vi "BRig_RT__Case_Exp__State_initTrial__v10.vi"(0 "input_dataCurrent":u16[](array[numeric]), 9 "input_dataBlock":u16[][](array[numeric]), 11 "input_dataTrial":u16[][](array[numeric]), 12 "input_dataExp":u16[](array[numeric])) -> (1 "output_iTrial":u16, 2 "output_nTrial":u16, 3 "output_SolenoidReward":bool, 4 "output_dataCurrent":u16[](array[numeric]), 10 "output_dataBlock":u16[][](array[numeric]), 15 "output_dataTrial":u16[][](array[numeric]))   [LabVIEW 2014]
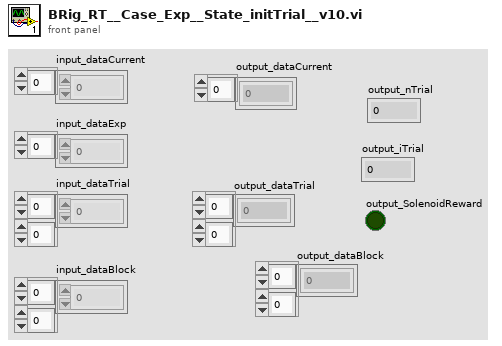
[diagram p1: front panel]
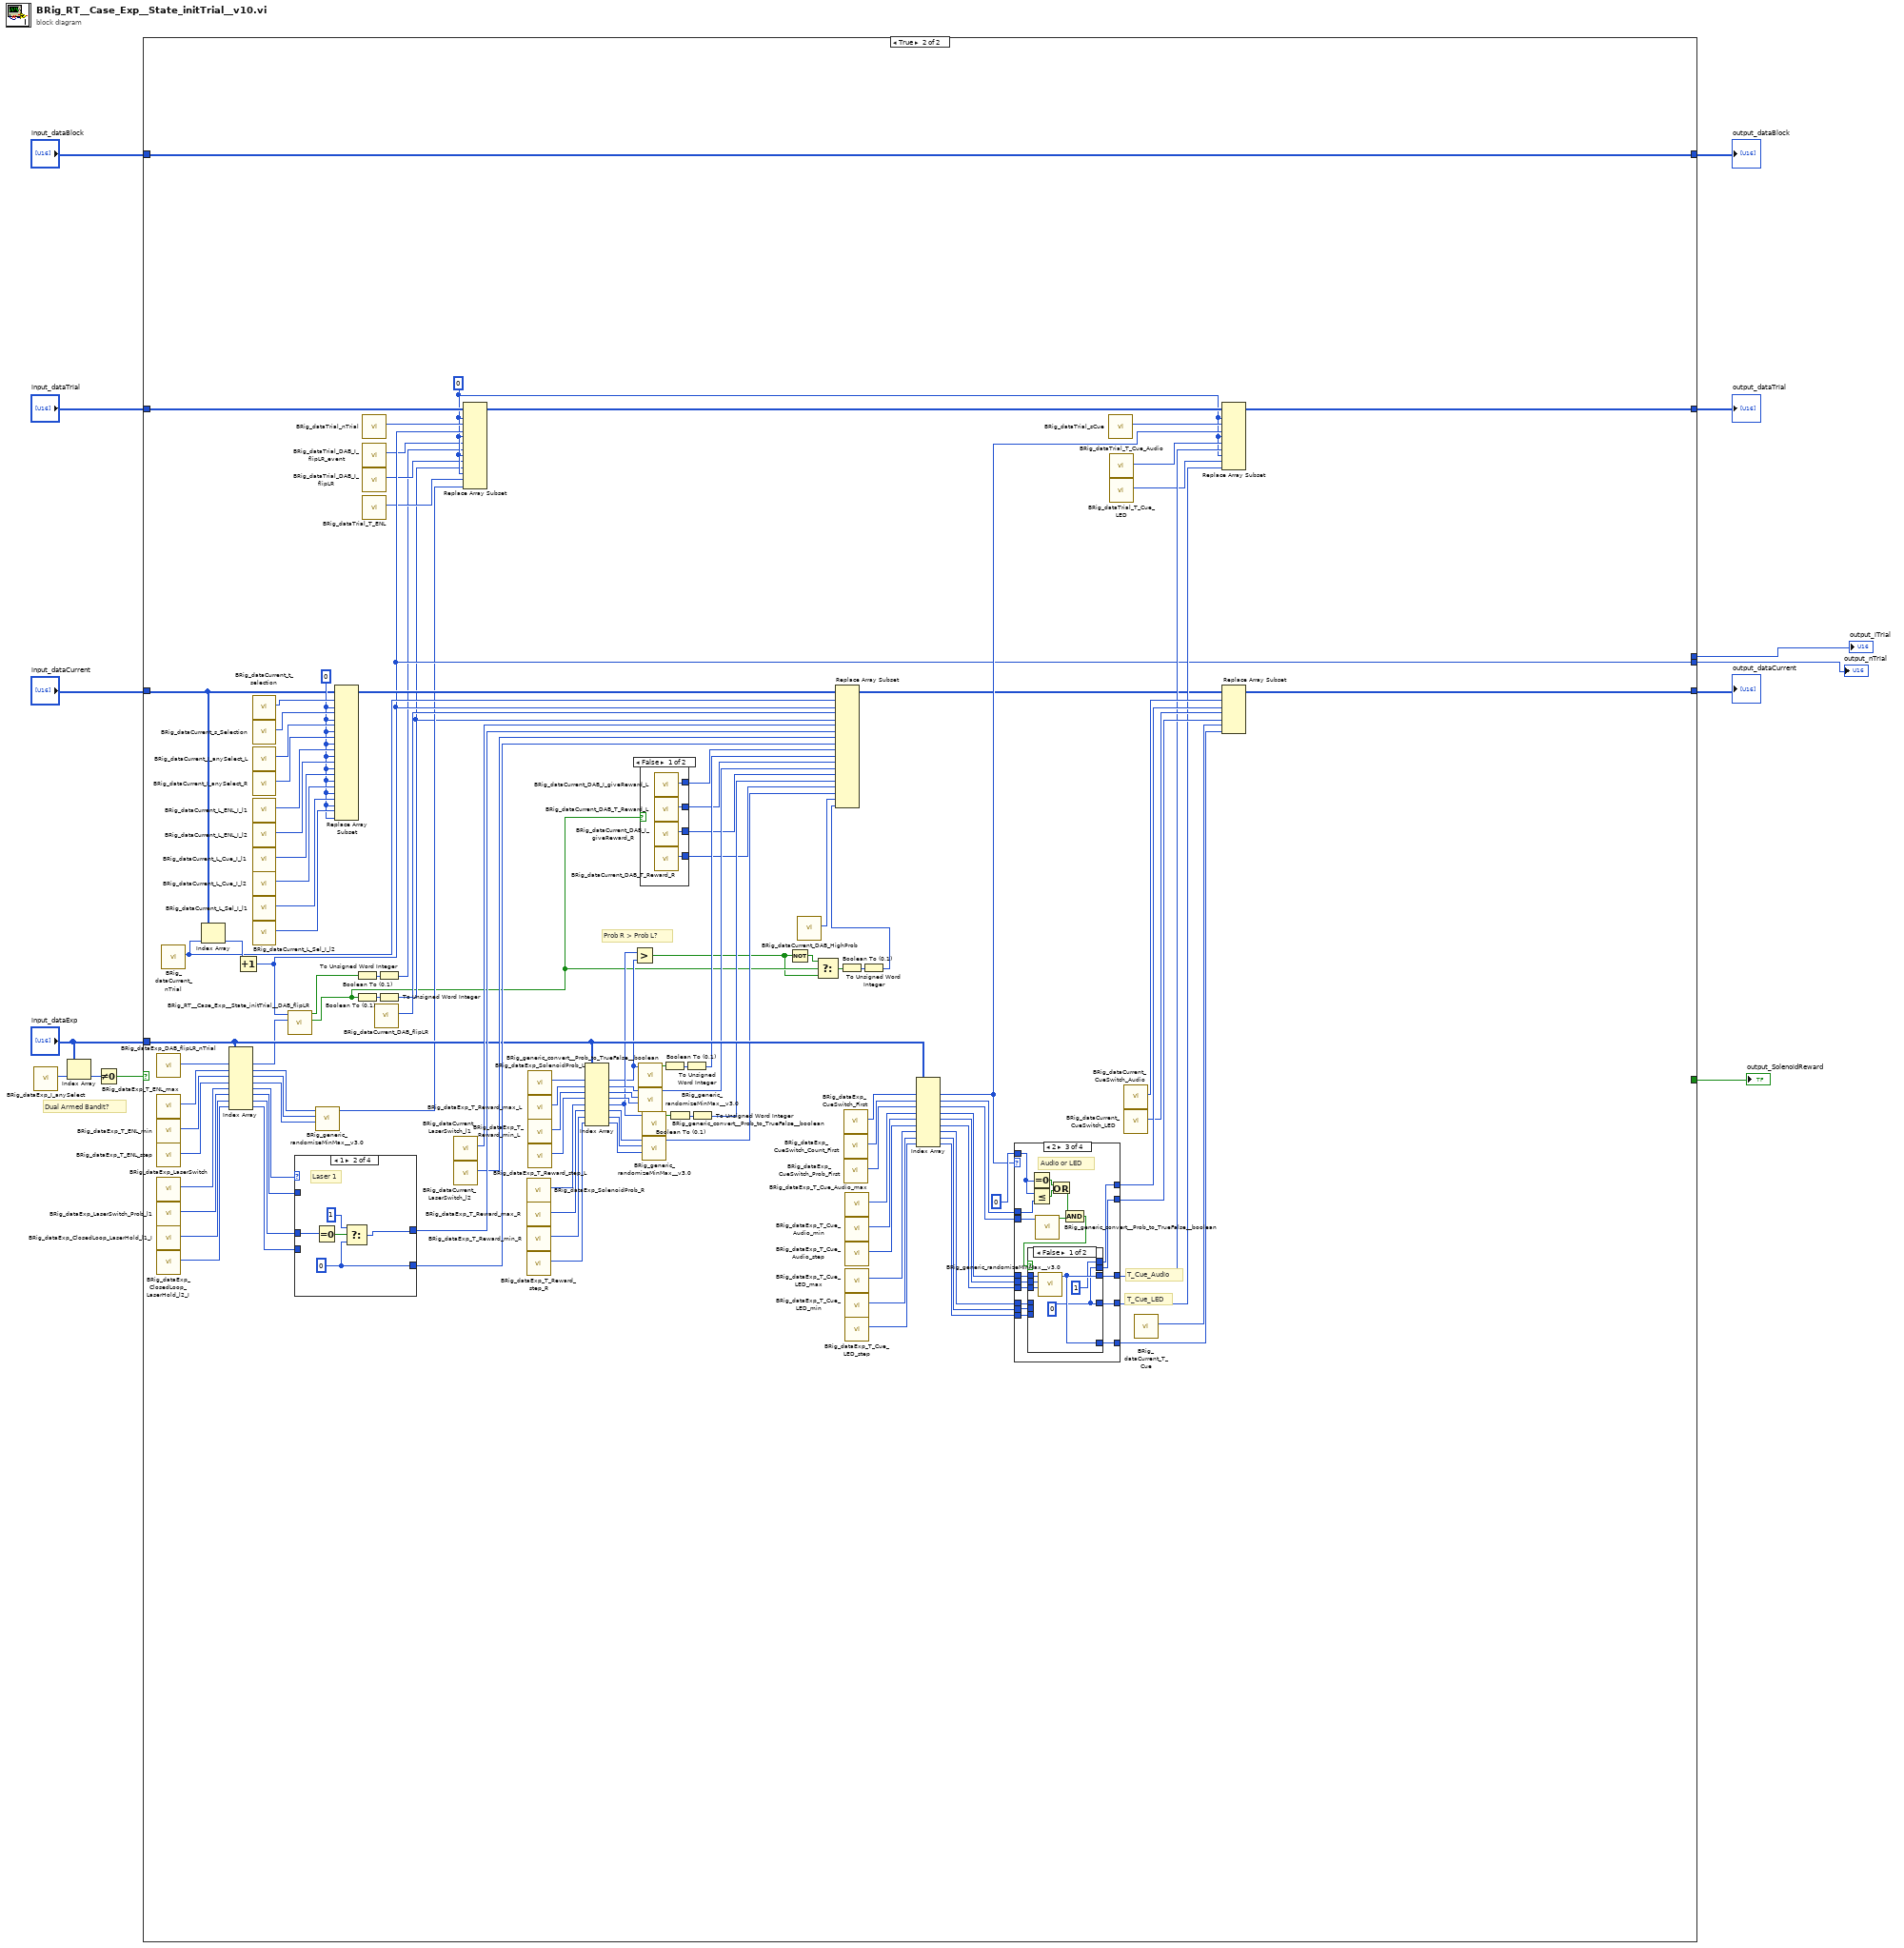
[diagram p0: block diagram]
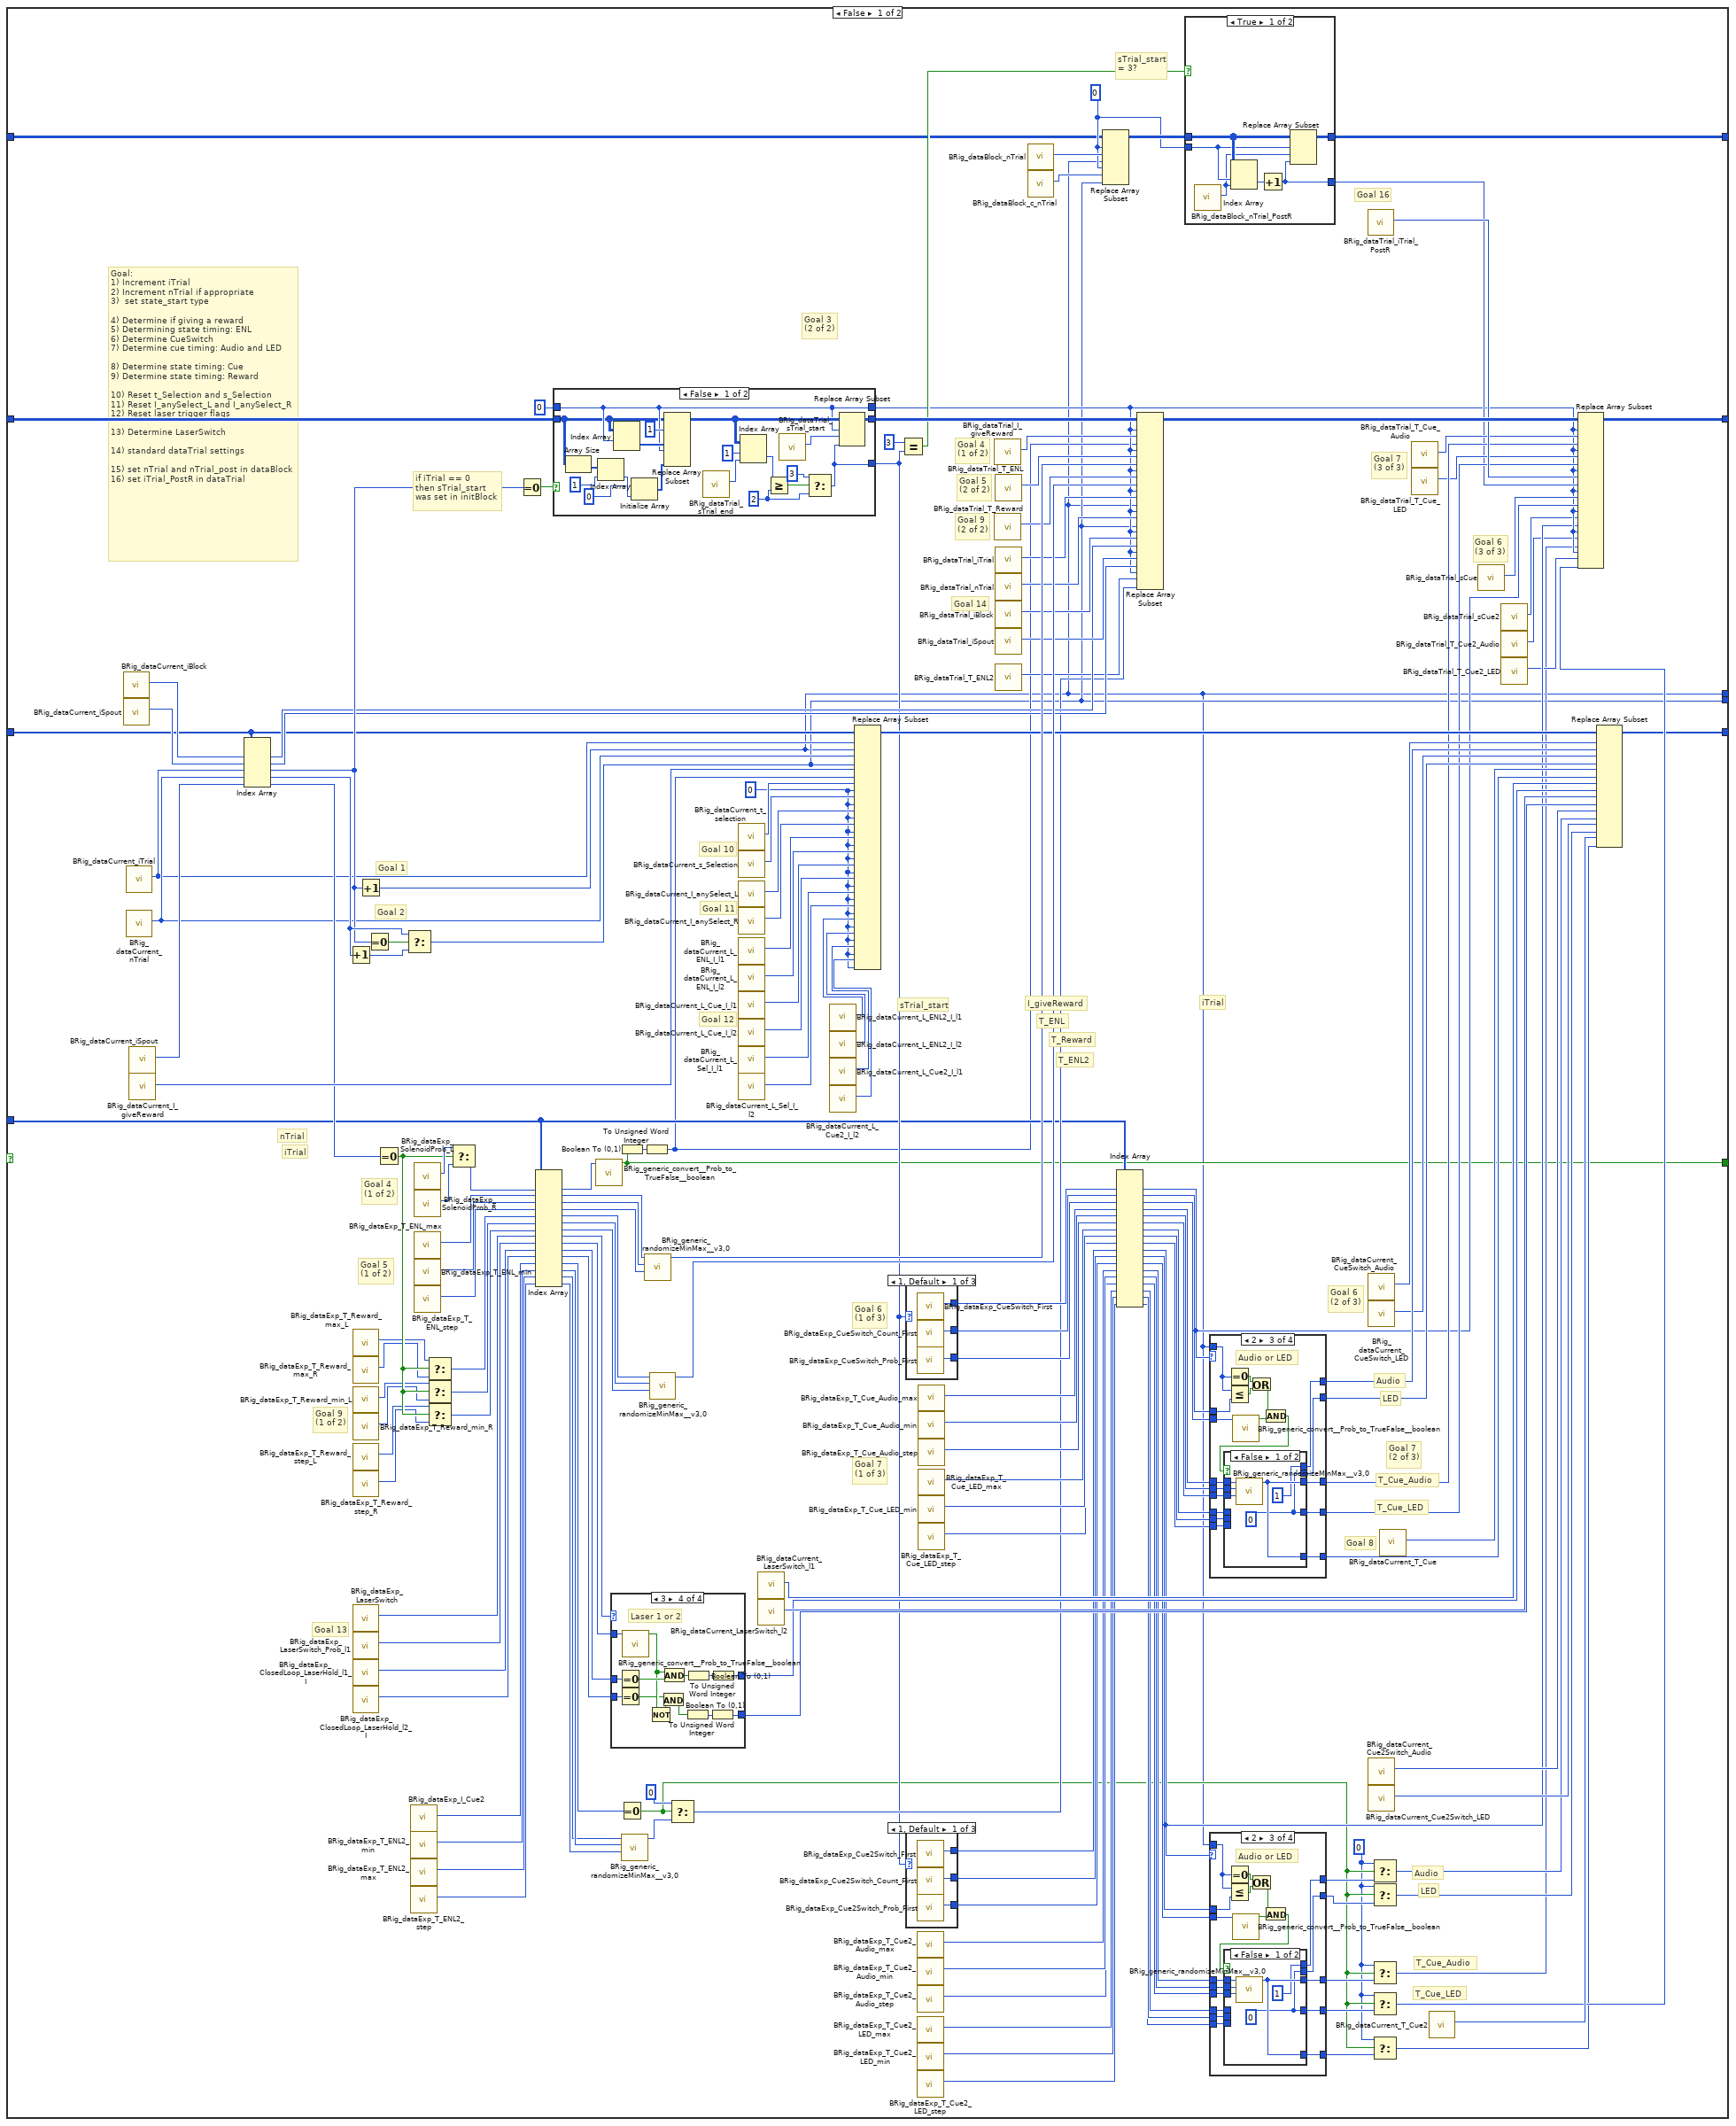
[diagram p2: hidden frame]
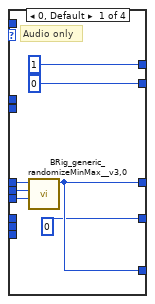
[diagram p3: hidden frame]
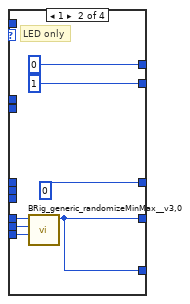
[diagram p4: hidden frame]
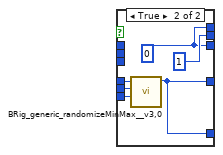
[diagram p5: hidden frame]
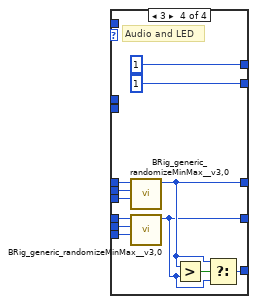
[diagram p6: hidden frame]
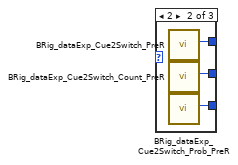
[diagram p7: hidden frame]
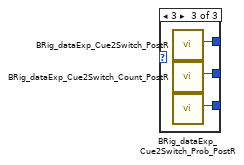
[diagram p8: hidden frame]
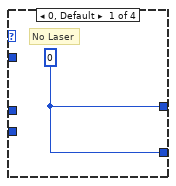
[diagram p10: hidden frame]
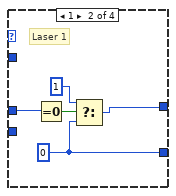
[diagram p11: hidden frame]
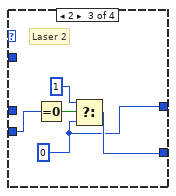
[diagram p12: hidden frame]
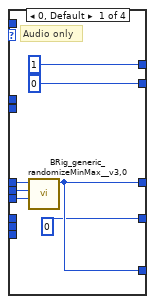
[diagram p13: hidden frame]
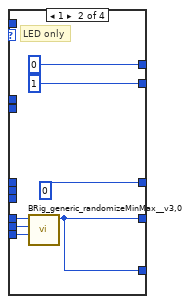
[diagram p14: hidden frame]
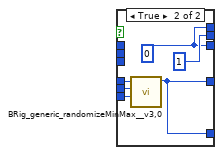
[diagram p15: hidden frame]
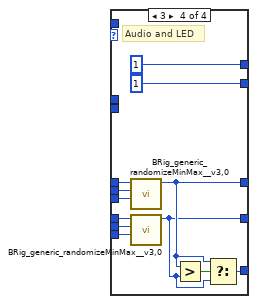
[diagram p16: hidden frame]
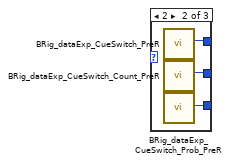
[diagram p17: hidden frame]
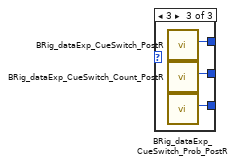
[diagram p18: hidden frame]
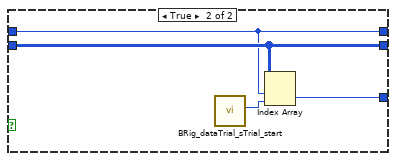
[diagram p19: hidden frame]
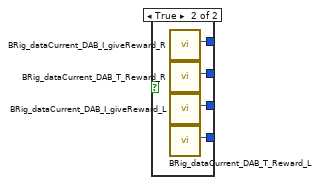
[diagram p20: hidden frame]
diagram:
  # "Dual Armed Bandit?"
  n1 = call "BRig_dataExp_I_anySelect.vi"() -> ("output_I_anySelect"=w13:i32)  [unwired: 11 in]
  n2 = Index Array(array="input_dataExp", index=w13) -> (element=w12:u16)
  n3 = Not Equal To 0?(x=w12) -> (x != 0?=w11:bool)
  n4 = case shown="True" w11 {
    tunnel: "input_dataExp" -> [w24 w421]
    tunnel: "input_dataCurrent" -> [w23 w430]
    tunnel: "input_dataTrial" -> [w22 w433]
    tunnel: "input_dataBlock" -> [w21 w494]
    tunnel: [w20 w494] -> w6
    tunnel: [w19 w447] -> w5
    tunnel: [w18 w448] -> w4
    tunnel: [w17 _] -> w3
    tunnel: [w15 w395] -> w2
    tunnel: [w14 _] -> w1
    frame False {
      w25 = u16 0 ("t")
      w83 = 0 ("disabled index (row)")
      w63 = u16 0 ("new element/subarray")
      # "T_Cue_LED"
      # "T_Cue_Audio"
      # "LED"
      # "Audio"
      # "T_ENL2"
      # "Goal 16"
      # "Goal 6\n(3 of 3)"
      # "iTrial"
      # "sTrial_start\n= 3?"
      # "nTrial"
      # "Goal 14"
      # "Goal 13"
      # "iTrial"
      # "Goal 8"
      # "Goal 7\n(3 of 3)"
      # "Goal 7\n(2 of 3)"
      # "Goal 7\n(1 of 3)"
      # "T_Cue_LED"
      # "T_Cue_Audio"
      # "I_giveReward"
      # "Goal 4\n(1 of 2)"
      # "T_Reward"
      # "Goal 9\n(2 of 2)"
      # "Goal 9\n(1 of 2)"
      # "Goal 12"
      # "Goal 11"
      # "Goal 10"
      # "T_ENL"
      # "sTrial_start"
      # "LED"
      # "Audio"
      # "Goal 6\n(2 of 3)"
      # "Goal 6\n(1 of 3)"
      # "Goal 3\n(2 of 2)"
      # "Goal 5\n(2 of 2)"
      # "Goal 5\n(1 of 2)"
      # "Goal 4\n(1 of 2)"
      # "if iTrial == 0\nthen sTrial_start\nwas set in initBlock"
      # "Goal 2"
      # "Goal 1"
      # "Goal:\n1) Increment iTrial\n2) Increment nTrial if appropriate\n3)  set state_start type\n\n4) Determine if giving a reward\n5) Determining state timing: ENL\n6) Determine CueSwitch\n7) Determine cue timing: Audio and LED\n\n8) Determine state timing: Cue\n9) Determine state timing: Reward\n\n10) Reset t_Selection and s_Selection\n11) Reset I_anySelect_L and I_anySelect_R\n12) Reset laser trigger flags\n\n13) Determine LaserSwitch\n\n14) standard dataTrial settings\n\n15) set nTrial and nTrial_post in dataBlock\n16) set iTrial_PostR in dataTrial"
      n5 = call "BRig_dataCurrent_iBlock.vi"() -> ("output_iBlock"=w99:i32)  [unwired: 11 in]
      n6 = call "BRig_dataCurrent_iSpout.vi"() -> ("output_iSpout"=w98:i32)  [unwired: 11 in]
      n7 = call "BRig_dataCurrent_iTrial.vi"() -> ("output_iTrial"=w80:i32)  [unwired: 11 in]
      n8 = call "BRig_dataCurrent_nTrial.vi"() -> ("output_nTrial"=w81:i32)  [unwired: 11 in]
      n9 = call "BRig_dataCurrent_iSpout.vi"() -> ("output_iSpout"=w90:i32)  [unwired: 11 in]
      n10 = call "BRig_dataCurrent_I_giveReward.vi"() -> ("output_I_giveReward"=w184:i32)  [unwired: 11 in]
      n11 = Index Array(array=w23, index #1=w99, index #2=w98, index #3=w80, index #4=w81, index #5=w90) -> (element #1=w108:u16, element #2=w107:u16, element #3=w121:u16, element #4=w188:u16, element #5=w89:u16)
      n12 = Increment(x=w188) -> (x+1=w187:u16)
      n13 = call "BRig_dataExp_T_Reward_max_L.vi"() -> ("output_T_Reward_max_L"=w152:i32)  [unwired: 11 in]
      n14 = call "BRig_dataExp_T_Reward_max_R.vi"() -> ("output_T_Reward_max_R"=w151:i32)  [unwired: 11 in]
      n15 = call "BRig_dataExp_T_Reward_min_L.vi"() -> ("output_Tcycle_Reward_min_L"=w150:i32)  [unwired: 11 in]
      n16 = call "BRig_dataExp_T_Reward_min_R.vi"() -> ("output_T_Reward_min_R"=w149:i32)  [unwired: 11 in]
      n17 = call "BRig_dataExp_T_Reward_step_L.vi"() -> ("output_T_Reward_step_L"=w148:i32)  [unwired: 11 in]
      n18 = call "BRig_dataExp_T_Reward_step_R.vi"() -> ("output_T_Reward_step_R"=w147:i32)  [unwired: 11 in]
      n19 = call "BRig_dataExp_LaserSwitch.vi"() -> ("output_LaserSwitch"=w120:i32)  [unwired: 11 in]
      n20 = call "BRig_dataExp_LaserSwitch_Prob_l1.vi"() -> ("output_LaserSwitch_Probability_L1"=w119:i32)  [unwired: 11 in]
      n21 = call "BRig_dataExp_ClosedLoop_LaserHold_l1_I.vi"() -> ("output_CloseLoop_LaserHold_l1_I"=w95:i32)  [unwired: 11 in]
      n22 = call "BRig_dataExp_ClosedLoop_LaserHold_l2_I.vi"() -> ("output_CloseLoop_LaserHold_l2_I"=w94:i32)  [unwired: 11 in]
      n23 = Increment(x=w121) -> (x+1=w14:u16)
      n24 = Equal To 0?(x=w121) -> (x = 0?=w186:bool)
      n25 = Equal To 0?(x=w89) -> (x = 0?=w153:bool)
      n26 = Select(t=w188, s=w186, f=w187) -> (s? t:f=w15:u16)
      n27 = call "BRig_dataExp_I_Cue2.vi"() -> ("output_I_Cue2"=w79:i32)  [unwired: 11 in]
      n28 = call "BRig_dataExp_T_ENL2_min.vi"() -> ("output_T_ENL2_min"=w78:i32)  [unwired: 11 in]
      n29 = call "BRig_dataExp_T_ENL2_max.vi"() -> ("output_T_ENL2_max"=w77:i32)  [unwired: 11 in]
      n30 = call "BRig_dataExp_T_ENL2_step.vi"() -> ("output_T_ENL2_step"=w76:i32)  [unwired: 11 in]
      n31 = call "BRig_dataExp_SolenoidProb_L.vi"() -> ("output_SolenoidProbability_L"=w183:i32)  [unwired: 11 in]
      n32 = call "BRig_dataExp_SolenoidProb_R.vi"() -> ("output_SolenoidProbability_R"=w182:i32)  [unwired: 11 in]
      n33 = call "BRig_dataExp_T_ENL_max.vi"() -> ("output_T_ENL_max"=w177:i32)  [unwired: 11 in]
      n34 = call "BRig_dataExp_T_ENL_min.vi"() -> ("output_T_ENL_min"=w178:i32)  [unwired: 11 in]
      n35 = call "BRig_dataExp_T_ENL_step.vi"() -> ("output_T_ENL_step"=w179:i32)  [unwired: 11 in]
      n36 = Select(t=w152, s=w153, f=w151) -> (s? t:f=w146:i32)
      n37 = Select(t=w150, s=w153, f=w149) -> (s? t:f=w145:i32)
      n38 = Select(t=w148, s=w153, f=w147) -> (s? t:f=w144:i32)
      n39 = Select(t=w183, s=w153, f=w182) -> (s? t:f=w181:i32)
      n40 = Equal To 0?(x=w121) -> (x = 0?=w185:bool)
      n41 = Index Array(array=w24, index #1=w181, index #2=w177, index #3=w178, index #4=w179, index #5=w146, index #6=w145, index #7=w144, index #8=w120, index #9=w119, index #10=w95, index #11=w94, index #12=w79, index #13=w78, index #14=w77, index #15=w76) -> (element #1=w180:u16, element #2=w176:u16, element #3=w175:u16, element #4=w174:u16, element #5=w143:u16, element #6=w142:u16, element #7=w141:u16, element #8=w118:u16, element #9=w117:u16, element #10=w93:u16, element #11=w92:u16, element #12=w73:u16, element #13=w72:u16, element #14=w71:u16, element #15=w70:u16)
      n42 = case shown="False" w185 {
        tunnel: w22 -> [w358 w375]
        tunnel: [w369 w375] -> w173
        tunnel: 0 -> [w359 w374]
        tunnel: [w359 w374] -> w37
        tunnel: [w365 w372] -> w62
        frame False {
          w366 = u16 2 ("y")
          n43 = Array Size(array=w358) -> (size(s)=w357:i32[])
          n44 = Index Array(array=w357, index=1) -> (element=w355:i32)
          n45 = Index Array(array=w358, index (row)=w359) -> (element=w362:u16[])  [unwired: 1 in]
          n46 = Initialize Array(u16 0 ("index"), w355) -> (w353:u16[])
          n47 = Replace Array Subset(array=w358, new element #1=w362, index (row) #1=1 ("index (row)"), new element #2=w353, index (row) #2=w359) -> (w360:u16[][])  [unwired: 2 in]
          n48 = call "BRig_dataTrial_sTrial_end.vi"() -> ("output_sTrial_end"=w371:i32)  [unwired: 11 in]
          n49 = Index Array(array=w360, index (row)=1 ("disabled index (row)"), index (col)=w371) -> (element=w370:u16)
          n50 = Greater Or Equal?(x=w370, y=w366) -> (x >= y?=w368:bool)
          n51 = call "BRig_dataTrial_sTrial_start.vi"() -> ("output_sTrial_start"=w364:i32)  [unwired: 11 in]
          n52 = Select(t=u16 3 ("y"), s=w368, f=w366) -> (s? t:f=w365:u16)
          n53 = Replace Array Subset(array=w360, new element=w365, index (row)=w359, index (col)=w364) -> (w369:u16[][])
        }
        frame True {
          n54 = call "BRig_dataTrial_sTrial_start.vi"() -> ("output_sTrial_start"=w373:i32)  [unwired: 11 in]
          n55 = Index Array(array=w375, index (row)=w374, index (col)=w373) -> (element=w372:u16)
        }
      }
      n56 = call "BRig_generic_convert__Prob_to_TrueFalse__boolean.vi"("input_probability_u16"=w180) -> ("output_TF"=w17:bool)  [unwired: 10 in]
      n57 = case shown="3" w118 {
        tunnel: [w263 w264 w269 w283] -> w115
        tunnel: [w263 w265 w270 w282] -> w114
        tunnel: w117 -> [_ _ _ w286]
        tunnel: w93 -> [_ w268 _ w281]
        tunnel: w92 -> [_ _ w271 w280]
        frame 0, Default {
          w263 = u16 0
          # "No Laser"
        }
        frame 1 {
          w265 = u16 0
          # "Laser 1"
          n58 = Equal To 0?(x=w268) -> (x = 0?=w267:bool)
          n59 = Select(t=u16 1, s=w267, f=w265) -> (s? t:f=w264:u16)
        }
        frame 2 {
          w269 = u16 0
          # "Laser 2"
          n60 = Equal To 0?(x=w271) -> (x = 0?=w273:bool)
          n61 = Select(t=u16 1, s=w273, f=w269) -> (s? t:f=w270:u16)
        }
        frame 3 {
          # "Laser 1 or 2"
          n62 = Equal To 0?(x=w281) -> (x = 0?=w279:bool)
          n63 = Equal To 0?(x=w280) -> (x = 0?=w275:bool)
          n64 = call "BRig_generic_convert__Prob_to_TrueFalse__boolean.vi"("input_probability_u16"=w286) -> ("output_TF"=w278:bool)  [unwired: 10 in]
          n65 = Not(x=w278) -> (.not. x?=w276:bool)
          n66 = And(x=w275, y=w276) -> (x .and. y?=w274:bool)
          n67 = And(x=w278, y=w279) -> (x .and. y?=w277:bool)
          n68 = Boolean To (0,1)(Boolean=w274) -> (0, 1=w285:i16)
          n69 = Boolean To (0,1)(Boolean=w277) -> (0, 1=w284:i16)
          n70 = To Unsigned Word Integer(number=w285) -> (unsigned 16bit integer=w282:u16)
          n71 = To Unsigned Word Integer(number=w284) -> (unsigned 16bit integer=w283:u16)
        }
      }
      n72 = Boolean To (0,1)(Boolean=w17) -> (0, 1=w189:i16)
      n73 = Equal To 0?(x=w73) -> (x = 0?=w26:bool)
      n74 = call "BRig_generic_randomizeMinMax__v3,0.vi"("Input_Increment"=w70, "Input_Min"=w72, "Input_Max"=w71) -> ("Output"=w75:u16)  [unwired: 8 in]
      n75 = To Unsigned Word Integer(number=w189) -> (unsigned 16bit integer=w16:u16)
      n76 = call "BRig_generic_randomizeMinMax__v3,0.vi"("Input_Increment"=w174, "Input_Min"=w175, "Input_Max"=w176) -> ("Output"=w171:u16)  [unwired: 8 in]
      n77 = call "BRig_generic_randomizeMinMax__v3,0.vi"("Input_Increment"=w141, "Input_Min"=w142, "Input_Max"=w143) -> ("Output"=w139:u16)  [unwired: 8 in]
      n78 = Select(t=u16 0, s=w26, f=w75) -> (s? t:f=w68:u16)
      n79 = call "BRig_dataCurrent_t_selection.vi"() -> ("output_t_selection"=w163:i32)  [unwired: 11 in]
      n80 = call "BRig_dataCurrent_s_Selection.vi"() -> ("output_s_Selection"=w162:i32)  [unwired: 11 in]
      n81 = call "BRig_dataCurrent_I_anySelect_L.vi"() -> ("output_IanySelect_L"=w161:i32)  [unwired: 11 in]
      n82 = call "BRig_dataCurrent_I_anySelect_R.vi"() -> ("output_IanySelect_R"=w160:i32)  [unwired: 11 in]
      n83 = call "BRig_dataCurrent_L_ENL_I_l1.vi"() -> ("output_L_ENL_I_l1"=w159:i32)  [unwired: 11 in]
      n84 = call "BRig_dataCurrent_L_ENL_I_l2.vi"() -> ("output_L_ENL_I_l2"=w158:i32)  [unwired: 11 in]
      n85 = call "BRig_dataCurrent_L_Cue_I_l1.vi"() -> ("output_L_Cue_I_l1"=w157:i32)  [unwired: 11 in]
      n86 = call "BRig_dataCurrent_L_Cue_I_l2.vi"() -> ("output_L_Cue_I_l2"=w156:i32)  [unwired: 11 in]
      n87 = call "BRig_dataCurrent_L_Sel_I_l1.vi"() -> ("output_L_Sel_I_l1"=w155:i32)  [unwired: 11 in]
      n88 = call "BRig_dataCurrent_L_Sel_I_l2.vi"() -> ("output_L_Sel_I_l2"=w154:i32)  [unwired: 11 in]
      n89 = call "BRig_dataCurrent_LaserSwitch_l1.vi"() -> ("output_LaserSwitch_l1"=w113:i32)  [unwired: 11 in]
      n90 = call "BRig_dataCurrent_LaserSwitch_l2.vi"() -> ("output_LaserSwitch_l2"=w116:i32)  [unwired: 11 in]
      n91 = call "BRig_dataCurrent_L_ENL2_I_l1.vi"() -> ("output_L_ENL2_I_l1"=w67:i32)  [unwired: 11 in]
      n92 = call "BRig_dataCurrent_L_ENL2_I_l2.vi"() -> ("output_L_ENL2_I_l2"=w66:i32)  [unwired: 11 in]
      n93 = call "BRig_dataCurrent_L_Cue2_I_l1.vi"() -> ("output_L_Cue2_I_l1"=w65:i32)  [unwired: 11 in]
      n94 = call "BRig_dataCurrent_L_Cue2_I_l2.vi"() -> ("output_L_Cue2_I_l2"=w64:i32)  [unwired: 11 in]
      n95 = Replace Array Subset(array=w23, new element #1=w14, index #1=w80, new element #2=w15, index #2=w81, new element #3=w16, index #3=w184, new element #4=w63, index #4=w163, new element #5=w63, index #5=w162, new element #6=w63, index #6=w161, new element #7=w63, index #7=w160, new element #8=w63, index #8=w159, new element #9=w63, index #9=w158, new element #10=w63, index #10=w157, new element #11=w63, index #11=w156, new element #12=w63, index #12=w155, new element #13=w63, index #13=w154, new element #14=w63, index #14=w67, new element #15=w63, index #15=w66, new element #16=w63, index #16=w65, new element #17=w63, index #17=w64) -> (w106:u16[])
      n96 = Equal?(x=u16 3 ("y"), y=w62) -> (x = y?=w84:bool)
      n97 = case shown="1, Default" w62 {
        tunnel: [w346 w347 w352] -> w170
        tunnel: [w345 w348 w351] -> w169
        tunnel: [w344 w349 w350] -> w168
        frame 1, Default {
          n98 = call "BRig_dataExp_CueSwitch_First.vi"() -> ("output_CueSwitch_First"=w346:i32)  [unwired: 11 in]
          n99 = call "BRig_dataExp_CueSwitch_Count_First.vi"() -> ("output_CueSwitch_Count_First"=w345:i32)  [unwired: 11 in]
          n100 = call "BRig_dataExp_CueSwitch_Prob_First.vi"() -> ("output_CueSwitch_Prob_First"=w344:i32)  [unwired: 11 in]
        }
        frame 2 {
          n101 = call "BRig_dataExp_CueSwitch_PreR.vi"() -> ("output_CueSwitch_PreR"=w347:i32)  [unwired: 11 in]
          n102 = call "BRig_dataExp_CueSwitch_Count_PreR.vi"() -> ("output_CueSwitch_Count_PreR"=w348:i32)  [unwired: 11 in]
          n103 = call "BRig_dataExp_CueSwitch_Prob_PreR.vi"() -> ("output_CueSwitch_Prob_PreR"=w349:i32)  [unwired: 11 in]
        }
        frame 3 {
          n104 = call "BRig_dataExp_CueSwitch_PostR.vi"() -> ("output_CueSwitch_PostR"=w352:i32)  [unwired: 11 in]
          n105 = call "BRig_dataExp_CueSwitch_Count_PostR.vi"() -> ("output_CueSwitch_Count_PostR"=w351:i32)  [unwired: 11 in]
          n106 = call "BRig_dataExp_CueSwitch_Prob_PostR.vi"() -> ("output_CueSwitch_Prob_PostR"=w350:i32)  [unwired: 11 in]
        }
      }
      n107 = case shown="1, Default" w62 {
        tunnel: [w249 w252 w255] -> w61
        tunnel: [w248 w251 w254] -> w60
        tunnel: [w247 w250 w253] -> w59
        frame 1, Default {
          n108 = call "BRig_dataExp_Cue2Switch_First.vi"() -> ("output_Cue2Switch_First"=w249:i32)  [unwired: 11 in]
          n109 = call "BRig_dataExp_Cue2Switch_Count_First.vi"() -> ("output_Cue2Switch_Count_First"=w248:i32)  [unwired: 11 in]
          n110 = call "BRig_dataExp_Cue2Switch_Prob_First.vi"() -> ("output_Cue2Switch_Prob_First"=w247:i32)  [unwired: 11 in]
        }
        frame 2 {
          n111 = call "BRig_dataExp_Cue2Switch_PreR.vi"() -> ("output_Cue2Switch_PreR"=w252:i32)  [unwired: 11 in]
          n112 = call "BRig_dataExp_Cue2Switch_Count_PreR.vi"() -> ("output_Cue2Switch_Count_PreR"=w251:i32)  [unwired: 11 in]
          n113 = call "BRig_dataExp_Cue2Switch_Prob_PreR.vi"() -> ("output_Cue2Switch_Prob_PreR"=w250:i32)  [unwired: 11 in]
        }
        frame 3 {
          n114 = call "BRig_dataExp_Cue2Switch_PostR.vi"() -> ("output_Cue2Switch_PostR"=w255:i32)  [unwired: 11 in]
          n115 = call "BRig_dataExp_Cue2Switch_Count_PostR.vi"() -> ("output_Cue2Switch_Count_PostR"=w254:i32)  [unwired: 11 in]
          n116 = call "BRig_dataExp_Cue2Switch_Prob_PostR.vi"() -> ("output_Cue2Switch_Prob_PostR"=w253:i32)  [unwired: 11 in]
        }
      }
      n117 = call "BRig_dataExp_T_Cue2_Audio_max.vi"() -> ("output_T_Cue2_Audio_max"=w58:i32)  [unwired: 11 in]
      n118 = call "BRig_dataExp_T_Cue2_Audio_min.vi"() -> ("output_T_Cue2_Audio_min"=w57:i32)  [unwired: 11 in]
      n119 = call "BRig_dataExp_T_Cue2_Audio_step.vi"() -> ("output_T_Cue2_Audio_step"=w56:i32)  [unwired: 11 in]
      n120 = call "BRig_dataExp_T_Cue2_LED_max.vi"() -> ("output_T_Cue2_LED_max"=w55:i32)  [unwired: 11 in]
      n121 = call "BRig_dataExp_T_Cue2_LED_min.vi"() -> ("output_T_Cue2_LED_min"=w54:i32)  [unwired: 11 in]
      n122 = call "BRig_dataExp_T_Cue2_LED_step.vi"() -> ("output_T_Cue2_LED_step"=w53:i32)  [unwired: 11 in]
      n123 = call "BRig_dataExp_T_Cue_Audio_max.vi"() -> ("output_T_Cue_Audio_max"=w137:i32)  [unwired: 11 in]
      n124 = call "BRig_dataExp_T_Cue_Audio_min.vi"() -> ("output_T_Cue_Audio_min"=w136:i32)  [unwired: 11 in]
      n125 = call "BRig_dataExp_T_Cue_Audio_step.vi"() -> ("output_T_Cue_Audio_step"=w135:i32)  [unwired: 11 in]
      n126 = call "BRig_dataExp_T_Cue_LED_max.vi"() -> ("output_T_Cue_LED_max"=w134:i32)  [unwired: 11 in]
      n127 = call "BRig_dataExp_T_Cue_LED_min.vi"() -> ("output_T_Cue_LED_min"=w133:i32)  [unwired: 11 in]
      n128 = call "BRig_dataExp_T_Cue_LED_step.vi"() -> ("output_T_Cue_LED_step"=w132:i32)  [unwired: 11 in]
      n129 = call "BRig_dataTrial_I_giveReward.vi"() -> ("output_I_giveReward"=w138:i32)  [unwired: 11 in]
      n130 = call "BRig_dataTrial_T_Reward.vi"() -> ("output_T_Reward"=w140:i32)  [unwired: 11 in]
      n131 = call "BRig_dataTrial_T_ENL.vi"() -> ("output_T_ENL"=w172:i32)  [unwired: 11 in]
      n132 = call "BRig_dataTrial_iTrial.vi"() -> ("output_iTrial"=w112:i32)  [unwired: 11 in]
      n133 = call "BRig_dataTrial_nTrial.vi"() -> ("output_nTrial"=w111:i32)  [unwired: 11 in]
      n134 = call "BRig_dataTrial_iBlock.vi"() -> ("output_iBlock"=w110:i32)  [unwired: 11 in]
      n135 = call "BRig_dataTrial_iSpout.vi"() -> ("output_iSpout"=w109:i32)  [unwired: 11 in]
      n136 = call "BRig_dataTrial_T_ENL2.vi"() -> ("output_T_ENL2"=w69:i32)  [unwired: 11 in]
      n137 = call "BRig_dataBlock_nTrial.vi"() -> ("output_nTrial"=w86:i32)  [unwired: 11 in]
      n138 = call "BRig_dataBlock_c_nTrial.vi"() -> ("output_c_nTrial"=w85:i32)  [unwired: 11 in]
      n139 = Replace Array Subset(array=w21, new element #1=w14, index (row) #1=w83, index (col) #1=w86, new element #2=w15, index (row) #2=w83, index (col) #2=w85) -> (w87:u16[][])
      n140 = Index Array(array=w24, index #1=w170, index #2=w169, index #3=w168, index #4=w137, index #5=w136, index #6=w135, index #7=w134, index #8=w133, index #9=w132, index #10=w61, index #11=w60, index #12=w59, index #13=w58, index #14=w57, index #15=w56, index #16=w55, index #17=w54, index #18=w53) -> (element #1=w96:u16, element #2=w131:u16, element #3=w130:u16, element #4=w129:u16, element #5=w128:u16, element #6=w127:u16, element #7=w126:u16, element #8=w125:u16, element #9=w124:u16, element #10=w36:u16, element #11=w52:u16, element #12=w51:u16, element #13=w50:u16, element #14=w49:u16, element #15=w48:u16, element #16=w47:u16, element #17=w46:u16, element #18=w45:u16)
      n141 = Replace Array Subset(array=w173, new element #1=w16, index (row) #1=w37, index (col) #1=w138, new element #2=w171, index (row) #2=w37, index (col) #2=w172, new element #3=w139, index (row) #3=w37, index (col) #3=w140, new element #4=w14, index (row) #4=w37, index (col) #4=w112, new element #5=w15, index (row) #5=w37, index (col) #5=w111, new element #6=w108, index (row) #6=w37, index (col) #6=w110, new element #7=w107, index (row) #7=w37, index (col) #7=w109, new element #8=w68, index (row) #8=w37, index (col) #8=w69) -> (w105:u16[][])
      n142 = case shown="True" w84 {
        tunnel: w87 -> [w261 w262]
        tunnel: [w259 w262] -> w20
        tunnel: [w256 _] -> w82
        tunnel: w83 -> [w258 _]
        frame True {
          n143 = call "BRig_dataBlock_nTrial_PostR.vi"() -> ("output_nTrial_PostR"=w257:i32)  [unwired: 11 in]
          n144 = Index Array(array=w261, index (row)=w258, index (col)=w257) -> (element=w260:u16)
          n145 = Increment(x=w260) -> (x+1=w256:u16)
          n146 = Replace Array Subset(array=w261, new element=w256, index (row)=w258, index (col)=w257) -> (w259:u16[][])
        }
        frame False {
        }
      }
      n147 = case shown="2" w96 {
        tunnel: [u16 1 u16 0 w305 u16 1] -> w166
        tunnel: [u16 0 u16 1 w304 u16 1] -> w164
        tunnel: w131 -> [_ _ w318 _]
        tunnel: w130 -> [_ _ w315 _]
        tunnel: w129 -> [w291 _ w311 w341]
        tunnel: w128 -> [w290 _ w310 w340]
        tunnel: w127 -> [w289 _ w309 w339]
        tunnel: w126 -> [_ w298 w303 w338]
        tunnel: w125 -> [_ w297 w302 w337]
        tunnel: w124 -> [_ w296 w301 w336]
        tunnel: [w288 u16 0 ("Output") w308 w334] -> w103
        tunnel: [u16 0 ("Output") w295 w306 w333] -> w102
        tunnel: [w288 w295 w307 w332] -> w122
        tunnel: w14 -> [_ _ w319 _]
        frame 0, Default {
          # "Audio only"
          n148 = call "BRig_generic_randomizeMinMax__v3,0.vi"("Input_Increment"=w289, "Input_Min"=w290, "Input_Max"=w291) -> ("Output"=w288:u16)  [unwired: 8 in]
        }
        frame 1 {
          # "LED only"
          n149 = call "BRig_generic_randomizeMinMax__v3,0.vi"("Input_Increment"=w296, "Input_Min"=w297, "Input_Max"=w298) -> ("Output"=w295:u16)  [unwired: 8 in]
        }
        frame 2 {
          # "Audio or LED"
          n150 = Equal To 0?(x=w319) -> (x = 0?=w317:bool)
          n151 = Less Or Equal?(x=w319, y=w318) -> (x <= y?=w316:bool)
          n152 = call "BRig_generic_convert__Prob_to_TrueFalse__boolean.vi"("input_probability_u16"=w315) -> ("output_TF"=w314:bool)  [unwired: 10 in]
          n153 = Or(x=w317, y=w316) -> (x .or. y?=w313:bool)
          n154 = And(x=w313, y=w314) -> (x .and. y?=w312:bool)
          n155 = case shown="False" w312 {
            tunnel: w311 -> [w325 _]
            tunnel: w310 -> [w324 _]
            tunnel: w309 -> [w323 _]
            tunnel: [w322 w326] -> w308
            tunnel: [w322 w328] -> w307
            tunnel: [w320 w328] -> w306
            tunnel: [u16 1 w326] -> w305
            tunnel: [w320 u16 1] -> w304
            tunnel: w303 -> [_ w331]
            tunnel: w302 -> [_ w330]
            tunnel: w301 -> [_ w329]
            frame False {
              w320 = u16 0
              n156 = call "BRig_generic_randomizeMinMax__v3,0.vi"("Input_Increment"=w323, "Input_Min"=w324, "Input_Max"=w325) -> ("Output"=w322:u16)  [unwired: 8 in]
            }
            frame True {
              w326 = u16 0
              n157 = call "BRig_generic_randomizeMinMax__v3,0.vi"("Input_Increment"=w329, "Input_Min"=w330, "Input_Max"=w331) -> ("Output"=w328:u16)  [unwired: 8 in]
            }
          }
        }
        frame 3 {
          # "Audio and LED"
          n158 = call "BRig_generic_randomizeMinMax__v3,0.vi"("Input_Increment"=w339, "Input_Min"=w340, "Input_Max"=w341) -> ("Output"=w334:u16)  [unwired: 8 in]
          n159 = call "BRig_generic_randomizeMinMax__v3,0.vi"("Input_Increment"=w336, "Input_Min"=w337, "Input_Max"=w338) -> ("Output"=w333:u16)  [unwired: 8 in]
          n160 = Greater?(x=w334, y=w333) -> (0:w335:bool)
          n161 = Select(t=w334, s=w335, f=w333) -> (s? t:f=w332:u16)
        }
      }
      n162 = case shown="2" w36 {
        tunnel: [u16 1 u16 0 w208 u16 1] -> w43
        tunnel: [u16 0 u16 1 w207 u16 1] -> w44
        tunnel: w52 -> [_ _ w221 _]
        tunnel: w51 -> [_ _ w218 _]
        tunnel: w50 -> [w194 _ w214 w244]
        tunnel: w49 -> [w193 _ w213 w243]
        tunnel: w48 -> [w192 _ w212 w242]
        tunnel: w47 -> [_ w201 w206 w241]
        tunnel: w46 -> [_ w200 w205 w240]
        tunnel: w45 -> [_ w199 w204 w239]
        tunnel: [w191 u16 0 ("Output") w211 w237] -> w32
        tunnel: [u16 0 ("Output") w198 w209 w236] -> w30
        tunnel: [w191 w198 w210 w235] -> w28
        tunnel: w14 -> [_ _ w222 _]
        frame 0, Default {
          # "Audio only"
          n163 = call "BRig_generic_randomizeMinMax__v3,0.vi"("Input_Increment"=w192, "Input_Min"=w193, "Input_Max"=w194) -> ("Output"=w191:u16)  [unwired: 8 in]
        }
        frame 1 {
          # "LED only"
          n164 = call "BRig_generic_randomizeMinMax__v3,0.vi"("Input_Increment"=w199, "Input_Min"=w200, "Input_Max"=w201) -> ("Output"=w198:u16)  [unwired: 8 in]
        }
        frame 2 {
          # "Audio or LED"
          n165 = Equal To 0?(x=w222) -> (x = 0?=w220:bool)
          n166 = Less Or Equal?(x=w222, y=w221) -> (x <= y?=w219:bool)
          n167 = call "BRig_generic_convert__Prob_to_TrueFalse__boolean.vi"("input_probability_u16"=w218) -> ("output_TF"=w217:bool)  [unwired: 10 in]
          n168 = Or(x=w220, y=w219) -> (x .or. y?=w216:bool)
          n169 = And(x=w216, y=w217) -> (x .and. y?=w215:bool)
          n170 = case shown="False" w215 {
            tunnel: w214 -> [w228 _]
            tunnel: w213 -> [w227 _]
            tunnel: w212 -> [w226 _]
            tunnel: [w225 w229] -> w211
            tunnel: [w225 w231] -> w210
            tunnel: [w223 w231] -> w209
            tunnel: [u16 1 w229] -> w208
            tunnel: [w223 u16 1] -> w207
            tunnel: w206 -> [_ w234]
            tunnel: w205 -> [_ w233]
            tunnel: w204 -> [_ w232]
            frame False {
              w223 = u16 0
              n171 = call "BRig_generic_randomizeMinMax__v3,0.vi"("Input_Increment"=w226, "Input_Min"=w227, "Input_Max"=w228) -> ("Output"=w225:u16)  [unwired: 8 in]
            }
            frame True {
              w229 = u16 0
              n172 = call "BRig_generic_randomizeMinMax__v3,0.vi"("Input_Increment"=w232, "Input_Min"=w233, "Input_Max"=w234) -> ("Output"=w231:u16)  [unwired: 8 in]
            }
          }
        }
        frame 3 {
          # "Audio and LED"
          n173 = call "BRig_generic_randomizeMinMax__v3,0.vi"("Input_Increment"=w242, "Input_Min"=w243, "Input_Max"=w244) -> ("Output"=w237:u16)  [unwired: 8 in]
          n174 = call "BRig_generic_randomizeMinMax__v3,0.vi"("Input_Increment"=w239, "Input_Min"=w240, "Input_Max"=w241) -> ("Output"=w236:u16)  [unwired: 8 in]
          n175 = Greater?(x=w237, y=w236) -> (0:w238:bool)
          n176 = Select(t=w237, s=w238, f=w236) -> (s? t:f=w235:u16)
        }
      }
      n177 = call "BRig_dataTrial_iTrial_PostR.vi"() -> ("output_iTrial_PostR"=w104:i32)  [unwired: 11 in]
      n178 = call "BRig_dataCurrent_CueSwitch_Audio.vi"() -> ("output_CueSwitch_Audio"=w167:i32)  [unwired: 11 in]
      n179 = call "BRig_dataCurrent_CueSwitch_LED.vi"() -> ("output_CueSwitch_LED"=w165:i32)  [unwired: 11 in]
      n180 = call "BRig_dataCurrent_Cue2Switch_Audio.vi"() -> ("output_Cue2Switch_Audio"=w42:i32)  [unwired: 11 in]
      n181 = call "BRig_dataCurrent_Cue2Switch_LED.vi"() -> ("output_Cue2Switch_LED"=w41:i32)  [unwired: 11 in]
      n182 = Select(t=w25, s=w26, f=w43) -> (s? t:f=w40:u16)
      n183 = Select(t=w25, s=w26, f=w44) -> (s? t:f=w39:u16)
      n184 = Select(t=w25, s=w26, f=w32) -> (s? t:f=w31:u16)
      n185 = Select(t=w25, s=w26, f=w30) -> (s? t:f=w29:u16)
      n186 = Select(t=w25, s=w26, f=w28) -> (s? t:f=w27:u16)
      n187 = call "BRig_dataCurrent_T_Cue.vi"() -> ("output_T_Cue"=w123:i32)  [unwired: 11 in]
      n188 = call "BRig_dataTrial_T_Cue_Audio.vi"() -> ("output_T_Cue_Audio"=w101:i32)  [unwired: 11 in]
      n189 = call "BRig_dataTrial_T_Cue_LED.vi"() -> ("output_T_Cue_LED"=w100:i32)  [unwired: 11 in]
      n190 = call "BRig_dataCurrent_T_Cue2.vi"() -> ("output_T_Cue2"=w38:i32)  [unwired: 11 in]
      n191 = call "BRig_dataTrial_sCue.vi"() -> ("output_sCue"=w97:i32)  [unwired: 11 in]
      n192 = call "BRig_dataTrial_sCue2.vi"() -> ("output_sCue2"=w35:i32)  [unwired: 11 in]
      n193 = call "BRig_dataTrial_T_Cue2_Audio.vi"() -> ("output_T_Cue2_Audio"=w34:i32)  [unwired: 11 in]
      n194 = call "BRig_dataTrial_T_Cue2_LED.vi"() -> ("output_T_Cue2_LED"=w33:i32)  [unwired: 11 in]
      n195 = Replace Array Subset(array=w105, new element #1=w103, index (row) #1=w37, index (col) #1=w101, new element #2=w102, index (row) #2=w37, index (col) #2=w100, new element #3=w82, index (row) #3=w37, index (col) #3=w104, new element #4=w96, index (row) #4=w37, index (col) #4=w97, new element #5=w36, index (row) #5=w37, index (col) #5=w35, new element #6=w31, index (row) #6=w37, index (col) #6=w34, new element #7=w29, index (row) #7=w37, index (col) #7=w33) -> (w19:u16[][])
      n196 = Replace Array Subset(array=w106, new element #1=w166, index #1=w167, new element #2=w164, index #2=w165, new element #3=w122, index #3=w123, new element #4=w115, index #4=w113, new element #5=w114, index #5=w116, new element #6=w40, index #6=w42, new element #7=w39, index #7=w41, new element #8=w27, index #8=w38) -> (w18:u16[])
    }
    frame True {
      w391 = 0
      w475 = u16 0 ("new element/subarray")
      # "Prob R > Prob L?"
      # "T_Cue_LED"
      # "T_Cue_Audio"
      n197 = call "BRig_dataExp_DAB_flipLR_nTrial.vi"() -> ("output_DAB_flipLR_nTrial"=w426:i32)  [unwired: 11 in]
      n198 = call "BRig_dataExp_T_ENL_max.vi"() -> ("output_T_ENL_max"=w492:i32)  [unwired: 11 in]
      n199 = call "BRig_dataExp_T_ENL_min.vi"() -> ("output_T_ENL_min"=w491:i32)  [unwired: 11 in]
      n200 = call "BRig_dataExp_T_ENL_step.vi"() -> ("output_T_ENL_step"=w490:i32)  [unwired: 11 in]
      n201 = call "BRig_dataExp_LaserSwitch.vi"() -> ("output_LaserSwitch"=w474:i32)  [unwired: 11 in]
      n202 = call "BRig_dataExp_LaserSwitch_Prob_l1.vi"() -> ("output_LaserSwitch_Probability_L1"=w473:i32)  [unwired: 11 in]
      n203 = call "BRig_dataExp_ClosedLoop_LaserHold_l1_I.vi"() -> ("output_CloseLoop_LaserHold_l1_I"=w472:i32)  [unwired: 11 in]
      n204 = call "BRig_dataExp_ClosedLoop_LaserHold_l2_I.vi"() -> ("output_CloseLoop_LaserHold_l2_I"=w471:i32)  [unwired: 11 in]
      n205 = call "BRig_dataCurrent_nTrial.vi"() -> ("output_nTrial"=w428:i32)  [unwired: 11 in]
      n206 = Index Array(array=w430, index=w428) -> (element=w493:u16)
      n207 = Index Array(array=w421, index #1=w426, index #2=w492, index #3=w491, index #4=w490, index #5=w474, index #6=w473, index #7=w472, index #8=w471) -> (element #1=w376:u16, element #2=w488:u16, element #3=w487:u16, element #4=w486:u16, element #5=w470:u16, element #6=w469:u16, element #7=w468:u16, element #8=w467:u16)
      n208 = Increment(x=w493) -> (x+1=w395:u16)
      n209 = call "BRig_dataCurrent_t_selection.vi"() -> ("output_t_selection"=w485:i32)  [unwired: 11 in]
      n210 = call "BRig_dataCurrent_s_Selection.vi"() -> ("output_s_Selection"=w484:i32)  [unwired: 11 in]
      n211 = call "BRig_dataCurrent_I_anySelect_L.vi"() -> ("output_IanySelect_L"=w483:i32)  [unwired: 11 in]
      n212 = call "BRig_dataCurrent_I_anySelect_R.vi"() -> ("output_IanySelect_R"=w482:i32)  [unwired: 11 in]
      n213 = call "BRig_dataCurrent_L_ENL_I_l1.vi"() -> ("output_L_ENL_I_l1"=w481:i32)  [unwired: 11 in]
      n214 = call "BRig_dataCurrent_L_ENL_I_l2.vi"() -> ("output_L_ENL_I_l2"=w480:i32)  [unwired: 11 in]
      n215 = call "BRig_dataCurrent_L_Cue_I_l1.vi"() -> ("output_L_Cue_I_l1"=w479:i32)  [unwired: 11 in]
      n216 = call "BRig_dataCurrent_L_Cue_I_l2.vi"() -> ("output_L_Cue_I_l2"=w478:i32)  [unwired: 11 in]
      n217 = call "BRig_dataCurrent_L_Sel_I_l1.vi"() -> ("output_L_Sel_I_l1"=w477:i32)  [unwired: 11 in]
      n218 = call "BRig_dataCurrent_L_Sel_I_l2.vi"() -> ("output_L_Sel_I_l2"=w476:i32)  [unwired: 11 in]
      n219 = call "BRig_RT__Case_Exp__State_initTrial__DAB_flipLR.vi"("input_DAB_flipLR_nTrial"=w376, "input_nTrial"=w395) -> ("output_switchedLR"=w382:bool, "output_flipOccurred"=w394:bool)  [unwired: 8 in]
      n220 = case shown="1" w470 {
        tunnel: [w560 w561 w566 w580] -> w424
        tunnel: [w560 w562 w567 w579] -> w422
        tunnel: w469 -> [_ _ _ w583]
        tunnel: w468 -> [_ w565 _ w578]
        tunnel: w467 -> [_ _ w568 w577]
        frame 0, Default {
          w560 = u16 0
          # "No Laser"
        }
        frame 1 {
          w562 = u16 0
          # "Laser 1"
          n221 = Equal To 0?(x=w565) -> (x = 0?=w564:bool)
          n222 = Select(t=u16 1, s=w564, f=w562) -> (s? t:f=w561:u16)
        }
        frame 2 {
          w566 = u16 0
          # "Laser 2"
          n223 = Equal To 0?(x=w568) -> (x = 0?=w570:bool)
          n224 = Select(t=u16 1, s=w570, f=w566) -> (s? t:f=w567:u16)
        }
        frame 3 {
          # "Laser 1 or 2"
          n225 = Equal To 0?(x=w578) -> (x = 0?=w576:bool)
          n226 = Equal To 0?(x=w577) -> (x = 0?=w572:bool)
          n227 = call "BRig_generic_convert__Prob_to_TrueFalse__boolean.vi"("input_probability_u16"=w583) -> ("output_TF"=w575:bool)  [unwired: 10 in]
          n228 = Not(x=w575) -> (.not. x?=w573:bool)
          n229 = And(x=w572, y=w573) -> (x .and. y?=w571:bool)
          n230 = And(x=w575, y=w576) -> (x .and. y?=w574:bool)
          n231 = Boolean To (0,1)(Boolean=w571) -> (0, 1=w582:i16)
          n232 = Boolean To (0,1)(Boolean=w574) -> (0, 1=w581:i16)
          n233 = To Unsigned Word Integer(number=w582) -> (unsigned 16bit integer=w579:u16)
          n234 = To Unsigned Word Integer(number=w581) -> (unsigned 16bit integer=w580:u16)
        }
      }
      n235 = call "BRig_generic_randomizeMinMax__v3,0.vi"("Input_Increment"=w486, "Input_Min"=w487, "Input_Max"=w488) -> ("Output"=w392:u16)  [unwired: 8 in]
      n236 = Replace Array Subset(array=w430, new element #1=w475, index #1=w485, new element #2=w475, index #2=w484, new element #3=w475, index #3=w483, new element #4=w475, index #4=w482, new element #5=w475, index #5=w481, new element #6=w475, index #6=w480, new element #7=w475, index #7=w479, new element #8=w475, index #8=w478, new element #9=w475, index #9=w477, new element #10=w475, index #10=w476) -> ()  [unwired: 1 out]
      n237 = Boolean To (0,1)(Boolean=w394) -> (0, 1=w396:i16)
      n238 = Boolean To (0,1)(Boolean=w382) -> (0, 1=w393:i16)
      n239 = call "BRig_dataTrial_nTrial.vi"() -> ("output_nTrial"=w431:i32)  [unwired: 11 in]
      n240 = call "BRig_dataTrial_DAB_I_flipLR_event.vi"() -> ("output_DAB_I_flipLR_event"=w389:i32)  [unwired: 11 in]
      n241 = call "BRig_dataTrial_DAB_I_flipLR.vi"() -> ("output_DAB_I_flipLR"=w388:i32)  [unwired: 11 in]
      n242 = call "BRig_dataTrial_T_ENL.vi"() -> ("output_T_ENL"=w390:i32)  [unwired: 11 in]
      n243 = call "BRig_dataCurrent_DAB_flipLR.vi"() -> ("output_DAB_flipLR"=w427:i32)  [unwired: 11 in]
      n244 = To Unsigned Word Integer(number=w396) -> (unsigned 16bit integer=w387:u16)
      n245 = To Unsigned Word Integer(number=w393) -> (unsigned 16bit integer=w386:u16)
      n246 = call "BRig_dataCurrent_LaserSwitch_l1.vi"() -> ("output_LaserSwitch_l1"=w425:i32)  [unwired: 11 in]
      n247 = call "BRig_dataCurrent_LaserSwitch_l2.vi"() -> ("output_LaserSwitch_l2"=w423:i32)  [unwired: 11 in]
      n248 = Replace Array Subset(array=w433, new element #1=w395, index (row) #1=w391, index (col) #1=w431, new element #2=w387, index (row) #2=w391, index (col) #2=w389, new element #3=w386, index (row) #3=w391, index (col) #3=w388, new element #4=w392, index (row) #4=w391, index (col) #4=w390) -> (w432:u16[][])
      n249 = call "BRig_dataExp_SolenoidProb_R.vi"() -> ("output_SolenoidProbability_R"=w416:i32)  [unwired: 11 in]
      n250 = call "BRig_dataExp_T_Reward_max_R.vi"() -> ("output_T_Reward_max_R"=w415:i32)  [unwired: 11 in]
      n251 = call "BRig_dataExp_T_Reward_min_R.vi"() -> ("output_T_Reward_min_R"=w414:i32)  [unwired: 11 in]
      n252 = call "BRig_dataExp_T_Reward_step_R.vi"() -> ("output_T_Reward_step_R"=w413:i32)  [unwired: 11 in]
      n253 = call "BRig_dataExp_SolenoidProb_L.vi"() -> ("output_SolenoidProbability_L"=w420:i32)  [unwired: 11 in]
      n254 = call "BRig_dataExp_T_Reward_max_L.vi"() -> ("output_T_Reward_max_L"=w419:i32)  [unwired: 11 in]
      n255 = call "BRig_dataExp_T_Reward_min_L.vi"() -> ("output_Tcycle_Reward_min_L"=w418:i32)  [unwired: 11 in]
      n256 = call "BRig_dataExp_T_Reward_step_L.vi"() -> ("output_T_Reward_step_L"=w417:i32)  [unwired: 11 in]
      n257 = Index Array(array=w421, index #1=w420, index #2=w419, index #3=w418, index #4=w417, index #5=w416, index #6=w415, index #7=w414, index #8=w413) -> (element #1=w384:u16, element #2=w412:u16, element #3=w411:u16, element #4=w410:u16, element #5=w385:u16, element #6=w409:u16, element #7=w408:u16, element #8=w407:u16)
      n258 = Greater?(x=w385, y=w384) -> (0:w381:bool)
      n259 = call "BRig_generic_convert__Prob_to_TrueFalse__boolean.vi"("input_probability_u16"=w384) -> ("output_TF"=w434:bool)  [unwired: 10 in]
      n260 = call "BRig_generic_randomizeMinMax__v3,0.vi"("Input_Increment"=w410, "Input_Min"=w411, "Input_Max"=w412) -> ("Output"=w401:u16)  [unwired: 8 in]
      n261 = case shown="False" w382 {
        tunnel: [w498 w501] -> w404
        tunnel: [w497 w500] -> w402
        tunnel: [w496 w499] -> w400
        tunnel: [w495 w502] -> w398
        frame False {
          n262 = call "BRig_dataCurrent_DAB_I_giveReward_L.vi"() -> ("output_DAB_I_giveReward_L"=w498:i32)  [unwired: 11 in]
          n263 = call "BRig_dataCurrent_DAB_T_Reward_L.vi"() -> ("output_DAB_T_Reward_L"=w497:i32)  [unwired: 11 in]
          n264 = call "BRig_dataCurrent_DAB_I_giveReward_R.vi"() -> ("output_DAB_I_giveReward_R"=w496:i32)  [unwired: 11 in]
          n265 = call "BRig_dataCurrent_DAB_T_Reward_R.vi"() -> ("output_DAB_T_Reward_R"=w495:i32)  [unwired: 11 in]
        }
        frame True {
          n266 = call "BRig_dataCurrent_DAB_I_giveReward_R.vi"() -> ("output_DAB_I_giveReward_R"=w501:i32)  [unwired: 11 in]
          n267 = call "BRig_dataCurrent_DAB_T_Reward_R.vi"() -> ("output_DAB_T_Reward_R"=w500:i32)  [unwired: 11 in]
          n268 = call "BRig_dataCurrent_DAB_I_giveReward_L.vi"() -> ("output_DAB_I_giveReward_L"=w499:i32)  [unwired: 11 in]
          n269 = call "BRig_dataCurrent_DAB_T_Reward_L.vi"() -> ("output_DAB_T_Reward_L"=w502:i32)  [unwired: 11 in]
        }
      }
      n270 = call "BRig_generic_convert__Prob_to_TrueFalse__boolean.vi"("input_probability_u16"=w385) -> ("output_TF"=w405:bool)  [unwired: 10 in]
      n271 = call "BRig_generic_randomizeMinMax__v3,0.vi"("Input_Increment"=w407, "Input_Min"=w408, "Input_Max"=w409) -> ("Output"=w397:u16)  [unwired: 8 in]
      n272 = Boolean To (0,1)(Boolean=w434) -> (0, 1=w489:i16)
      n273 = Boolean To (0,1)(Boolean=w405) -> (0, 1=w406:i16)
      n274 = To Unsigned Word Integer(number=w489) -> (unsigned 16bit integer=w403:u16)
      n275 = To Unsigned Word Integer(number=w406) -> (unsigned 16bit integer=w399:u16)
      n276 = Not(x=w381) -> (.not. x?=w383:bool)
      n277 = call "BRig_dataCurrent_DAB_HighProb.vi"() -> ("output_DAB_HighProb"=w378:i32)  [unwired: 11 in]
      n278 = Select(t=w383, s=w382, f=w381) -> (s? t:f=w379:bool)
      n279 = Boolean To (0,1)(Boolean=w379) -> (0, 1=w380:i16)
      n280 = call "BRig_dataExp_CueSwitch_First.vi"() -> ("output_CueSwitch_First"=w466:i32)  [unwired: 11 in]
      n281 = call "BRig_dataExp_CueSwitch_Count_First.vi"() -> ("output_CueSwitch_Count_First"=w465:i32)  [unwired: 11 in]
      n282 = call "BRig_dataExp_CueSwitch_Prob_First.vi"() -> ("output_CueSwitch_Prob_First"=w464:i32)  [unwired: 11 in]
      n283 = call "BRig_dataExp_T_Cue_Audio_max.vi"() -> ("output_T_Cue_Audio_max"=w463:i32)  [unwired: 11 in]
      n284 = call "BRig_dataExp_T_Cue_Audio_min.vi"() -> ("output_T_Cue_Audio_min"=w462:i32)  [unwired: 11 in]
      n285 = call "BRig_dataExp_T_Cue_Audio_step.vi"() -> ("output_T_Cue_Audio_step"=w461:i32)  [unwired: 11 in]
      n286 = call "BRig_dataExp_T_Cue_LED_max.vi"() -> ("output_T_Cue_LED_max"=w460:i32)  [unwired: 11 in]
      n287 = call "BRig_dataExp_T_Cue_LED_min.vi"() -> ("output_T_Cue_LED_min"=w459:i32)  [unwired: 11 in]
      n288 = call "BRig_dataExp_T_Cue_LED_step.vi"() -> ("output_T_Cue_LED_step"=w458:i32)  [unwired: 11 in]
      n289 = To Unsigned Word Integer(number=w380) -> (unsigned 16bit integer=w377:u16)
      n290 = Replace Array Subset(array=w430, new element #1=w395, index #1=w428, new element #2=w386, index #2=w427, new element #3=w424, index #3=w425, new element #4=w422, index #4=w423, new element #5=w403, index #5=w404, new element #6=w401, index #6=w402, new element #7=w399, index #7=w400, new element #8=w397, index #8=w398, new element #9=w377, index #9=w378) -> (w429:u16[])
      n291 = Index Array(array=w421, index #1=w466, index #2=w465, index #3=w464, index #4=w463, index #5=w462, index #6=w461, index #7=w460, index #8=w459, index #9=w458) -> (element #1=w441:u16, element #2=w456:u16, element #3=w455:u16, element #4=w454:u16, element #5=w453:u16, element #6=w452:u16, element #7=w451:u16, element #8=w450:u16, element #9=w449:u16)
      n292 = case shown="2" w441 {
        tunnel: [u16 1 u16 0 w521 u16 1] -> w445
        tunnel: [u16 0 u16 1 w520 u16 1] -> w443
        tunnel: w456 -> [_ _ w534 _]
        tunnel: w455 -> [_ _ w531 _]
        tunnel: w454 -> [w507 _ w527 w557]
        tunnel: w453 -> [w506 _ w526 w556]
        tunnel: w452 -> [w505 _ w525 w555]
        tunnel: w451 -> [_ w514 w519 w554]
        tunnel: w450 -> [_ w513 w518 w553]
        tunnel: w449 -> [_ w512 w517 w552]
        tunnel: [w504 u16 0 ("Output") w524 w550] -> w439
        tunnel: [u16 0 ("Output") w511 w522 w549] -> w437
        tunnel: [w504 w511 w523 w548] -> w435
        tunnel: u16 0 -> [_ _ w535 _]
        frame 0, Default {
          # "Audio only"
          n293 = call "BRig_generic_randomizeMinMax__v3,0.vi"("Input_Increment"=w505, "Input_Min"=w506, "Input_Max"=w507) -> ("Output"=w504:u16)  [unwired: 8 in]
        }
        frame 1 {
          # "LED only"
          n294 = call "BRig_generic_randomizeMinMax__v3,0.vi"("Input_Increment"=w512, "Input_Min"=w513, "Input_Max"=w514) -> ("Output"=w511:u16)  [unwired: 8 in]
        }
        frame 2 {
          # "Audio or LED"
          n295 = Equal To 0?(x=w535) -> (x = 0?=w533:bool)
          n296 = Less Or Equal?(x=w535, y=w534) -> (x <= y?=w532:bool)
          n297 = call "BRig_generic_convert__Prob_to_TrueFalse__boolean.vi"("input_probability_u16"=w531) -> ("output_TF"=w530:bool)  [unwired: 10 in]
          n298 = Or(x=w533, y=w532) -> (x .or. y?=w529:bool)
          n299 = And(x=w529, y=w530) -> (x .and. y?=w528:bool)
          n300 = case shown="False" w528 {
            tunnel: w527 -> [w541 _]
            tunnel: w526 -> [w540 _]
            tunnel: w525 -> [w539 _]
            tunnel: [w538 w542] -> w524
            tunnel: [w538 w544] -> w523
            tunnel: [w536 w544] -> w522
            tunnel: [u16 1 w542] -> w521
            tunnel: [w536 u16 1] -> w520
            tunnel: w519 -> [_ w547]
            tunnel: w518 -> [_ w546]
            tunnel: w517 -> [_ w545]
            frame False {
              w536 = u16 0
              n301 = call "BRig_generic_randomizeMinMax__v3,0.vi"("Input_Increment"=w539, "Input_Min"=w540, "Input_Max"=w541) -> ("Output"=w538:u16)  [unwired: 8 in]
            }
            frame True {
              w542 = u16 0
              n302 = call "BRig_generic_randomizeMinMax__v3,0.vi"("Input_Increment"=w545, "Input_Min"=w546, "Input_Max"=w547) -> ("Output"=w544:u16)  [unwired: 8 in]
            }
          }
        }
        frame 3 {
          # "Audio and LED"
          n303 = call "BRig_generic_randomizeMinMax__v3,0.vi"("Input_Increment"=w555, "Input_Min"=w556, "Input_Max"=w557) -> ("Output"=w550:u16)  [unwired: 8 in]
          n304 = call "BRig_generic_randomizeMinMax__v3,0.vi"("Input_Increment"=w552, "Input_Min"=w553, "Input_Max"=w554) -> ("Output"=w549:u16)  [unwired: 8 in]
          n305 = Greater?(x=w550, y=w549) -> (0:w551:bool)
          n306 = Select(t=w550, s=w551, f=w549) -> (s? t:f=w548:u16)
        }
      }
      n307 = call "BRig_dataTrial_sCue.vi"() -> ("output_sCue"=w442:i32)  [unwired: 11 in]
      n308 = call "BRig_dataTrial_T_Cue_Audio.vi"() -> ("output_T_Cue_Audio"=w440:i32)  [unwired: 11 in]
      n309 = call "BRig_dataTrial_T_Cue_LED.vi"() -> ("output_T_Cue_LED"=w438:i32)  [unwired: 11 in]
      n310 = call "BRig_dataCurrent_CueSwitch_Audio.vi"() -> ("output_CueSwitch_Audio"=w446:i32)  [unwired: 11 in]
      n311 = call "BRig_dataCurrent_CueSwitch_LED.vi"() -> ("output_CueSwitch_LED"=w444:i32)  [unwired: 11 in]
      n312 = call "BRig_dataCurrent_T_Cue.vi"() -> ("output_T_Cue"=w436:i32)  [unwired: 11 in]
      n313 = Replace Array Subset(array=w432, new element #1=w441, index (row) #1=w391, index (col) #1=w442, new element #2=w439, index (row) #2=w391, index (col) #2=w440, new element #3=w437, index (row) #3=w391, index (col) #3=w438) -> (w447:u16[][])
      n314 = Replace Array Subset(array=w429, new element #1=w445, index #1=w446, new element #2=w443, index #2=w444, new element #3=w435, index #3=w436) -> (w448:u16[])
    }
  }
  "output_dataBlock" <- w6
  "output_dataTrial" <- w5
  "output_dataCurrent" <- w4
  "output_SolenoidReward" <- w3
  "output_nTrial" <- w2
  "output_iTrial" <- w1
